vi "Grid Boundaries.vi"(1 "Grid":set{cdb}(c389)) -> (0 "Bounds":T1)   [LabVIEW 2020, in "AoC 2022.lvlib"]
uses:
  AoC 2022.lvlib
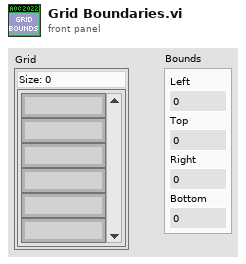
[diagram p1: front panel]
types:
  T1 = cluster{"Left":i16, "Top":i16, "Right":i16, "Bottom":i16}
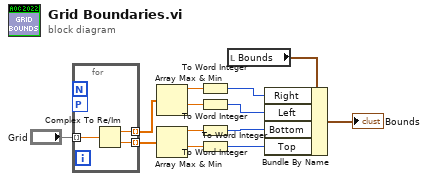
[diagram p0: block diagram]
diagram:
  n1 = for {
    tunnel: "Grid" -> [w16] mode=indexing
    tunnel: [w15] -> w12 mode=indexing
    tunnel: [w14] -> w13 mode=indexing
    workers-P: _ -> [_]
    n2 = Complex To Re/Im(x + iy=w16) -> (x=w15:dbl, y=w14:dbl)
  }
  n3 = Array Max & Min(array=w12) -> (max value=w10:dbl, min value=w9:dbl)  [unwired: 2 out]
  n4 = Array Max & Min(array=w13) -> (max value=w8:dbl, min value=w7:dbl)  [unwired: 2 out]
  n5 = To Word Integer(number=w10) -> (16bit integer=w5:i16)
  n6 = To Word Integer(number=w9) -> (16bit integer=w4:i16)
  n7 = To Word Integer(number=w8) -> (16bit integer=w2:i16)
  n8 = To Word Integer(number=w7) -> (16bit integer=w3:i16)
  n9 = local read "Bounds"() -> (w6:T1)
  n10 = Bundle By Name(cluster=w6, "Right"=w5, "Left"=w4, "Bottom"=w2, "Top"=w3) -> (→"Bounds":T1)
